vi "Initialize.vi"(9 "Column":i32, 10 "Row":i32, 11 "Starter in":refnum<class "Fortress.lvclass">) -> (3 "Starter out":refnum<class "Fortress.lvclass">)   [LabVIEW 2015, in "Fortress.lvclass"]
uses:
  Fortress.lvclass
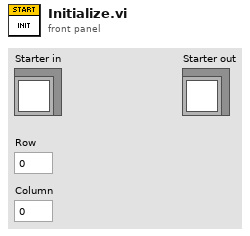
[diagram p1: front panel]
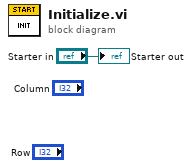
[diagram p0: block diagram]
diagram:
  "Starter out" <- "Starter in"
